vi "Error Converter (ErrCode or Status).vi"(8 "error in (no error)":errorcluster, 11 "error code":i32) -> (0 "error out":errorcluster)   [LabVIEW 2015, in "ESLSCDLL.lvlib"]
uses:
  ESLSCDLL.lvlib
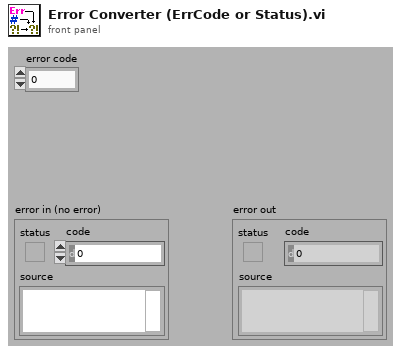
[diagram p1: front panel]
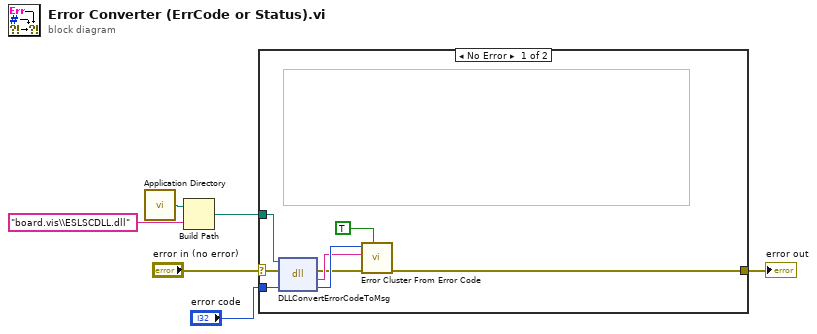
[diagram p0: block diagram]
diagram:
  n1 = call <vilib>:"Application Directory.vi"() -> ("Application Directory"=w3:path)
  n2 = Build Path(base path=w3, name or relative path="board.vis\\ESLSCDLL.dll") -> (appended path=w1:path)
  n3 = case shown="No Error" "error in (no error)" {
    selector: "error in (no error)" -> [w14 w15]
    tunnel: [w12 w15] -> w5
    tunnel: "error code" -> [w13 _]
    tunnel: w1 -> [w7 _]
    frame No Error {
      n4 = dll-call lib="C:/ENTW/PCIE/LV64/board.vis/ESLSCDLL.dll" fn="DLLConvertErrorCodeToMsg" ("lwlscdll.dll:DLLAboutDrv")(path in=w7, error in=w14, "status"=w13) -> (error out=w8:errorcluster, "msg"=w9:string, "status"=w10:i32)  [unwired: 1 in, 1 out]
      n5 = call <vilib>:"Error Cluster From Error Code.vi"("show call chain? (False)"=TRUE, "error in (no error)"=w8, "error message (\"\")"=w9, "error code (0)"=w10) -> ("error out"=w12:errorcluster)  [unwired: 5 in]
    }
    frame Error {
    }
  }
  "error out" <- w5
